vi "Login Response.vi"(8 "error in (no error)":errorcluster, 10 "success?":bool, 11 "[V] Login in":refnum<class "[V] Login.lvclass">) -> (0 "error out":errorcluster, 3 "[V] Login out":refnum<class "[V] Login.lvclass">)   [LabVIEW 2020, in "[V] Login.lvlib" / "[V] Login.lvclass"]
uses:
  [V] Login.lvclass
  [V] Login.lvclass/[V] Login.ctl
  <vilib>/ActorFramework/Message Enqueuer/Message Enqueuer.lvclass/Message Enqueuer.ctl
  <vilib>/ActorFramework/Message Enqueuer/Enqueue.vi
  <vilib>/ActorFramework/Stop Msg/Stop Msg.lvclass
  C:/Program Files (x86)/National Instruments/LabVIEW 2020/vi.lib/ActorFramework/Message/Message.lvclass
  <vilib>/ActorFramework/Message Priority Queue/Priority Enqueue.vi
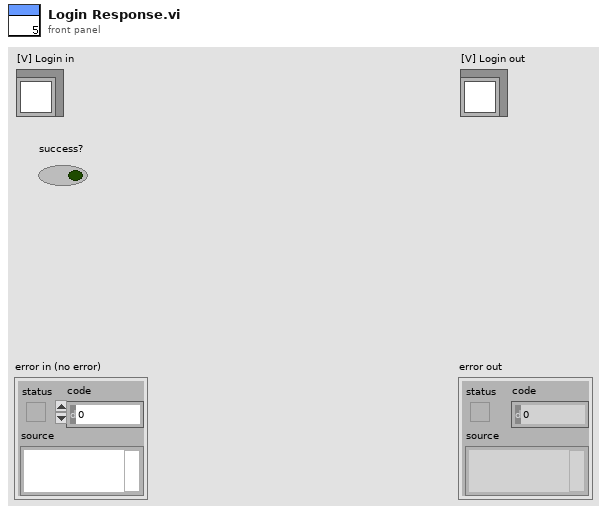
[diagram p1: front panel]
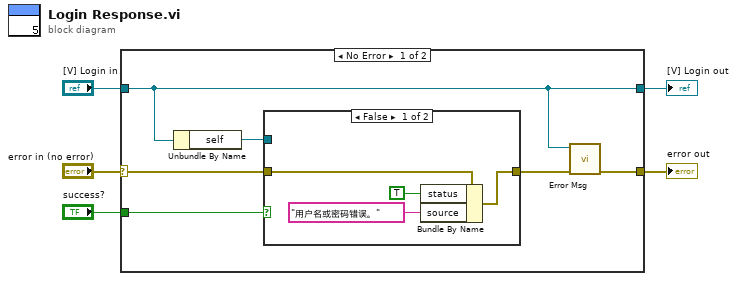
[diagram p0: block diagram]
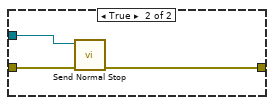
[diagram p2: hidden frame]
diagram:
  n1 = case shown="No Error" "error in (no error)" {
    selector: "error in (no error)" -> [w10 w20]
    tunnel: [w7 w20] -> w4
    tunnel: [w6 w19] -> w2
    tunnel: "[V] Login in" -> [w6 w19]
    tunnel: "success?" -> [w11 _]
    frame No Error {
      n2 = Unbundle By Name(w6) -> ("self"=w9:refnum<class "Message Enqueuer.lvclass">)
      n3 = case shown="False" w11 {
        tunnel: w10 -> [w15 w18]
        tunnel: w9 -> [_ w17]
        tunnel: [w12 w16] -> w8
        frame False {
          n4 = Bundle By Name(cluster=w15, "status"=TRUE, "source"="用户名或密码错误。") -> (w12:errorcluster)
        }
        frame True {
          n5 = call <vilib>:"Send Normal Stop.vi"("error in (no error)"=w18, "Message Enqueuer"=w17) -> ("error out"=w16:errorcluster)  [unwired: 9 in]
        }
      }
      n6 = call "Error Msg.vi"("error in (no error)"=w8, "[V] Login in"=w6) -> ("error out"=w7:errorcluster)  [unwired: 8 in, 1 out]
    }
    frame Error {
    }
  }
  "error out" <- w4
  "[V] Login out" <- w2
